vi "Launch Step Async.vi"(8 "error in (no error)":errorcluster, 10 "Step in":refnum<class "Step.lvclass">, 11 "Tester in":refnum<class "Tester.lvclass">) -> (0 "error out":errorcluster, 2 "Terminate":bool, 3 "Tester out":refnum<class "Tester.lvclass">)   [LabVIEW 2020, in "Tester.lvlib" / "Tester.lvclass"]
uses:
  Tester.lvclass
  Step/Step.lvclass
  Tester.lvclass/Tester.ctl
  Run Step Async.vi
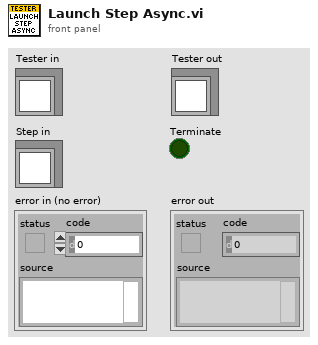
[diagram p1: front panel]
types:
  T1 = typedef "Tester.lvlib/Tester.lvclass/Execution Ref.ctl" = cluster{"Sequence":refnum<class "Sequence.lvclass">, "Step":i32, "Results":refnum<class "Results.lvclass">, "State":T2, "Run Step VI":refnum<vi>, "Abort":bool}
  T2 = typedef "Tester.lvlib/Tester.lvclass/State.ctl" = enum16{"Idle", "In Progress", "Completed"}
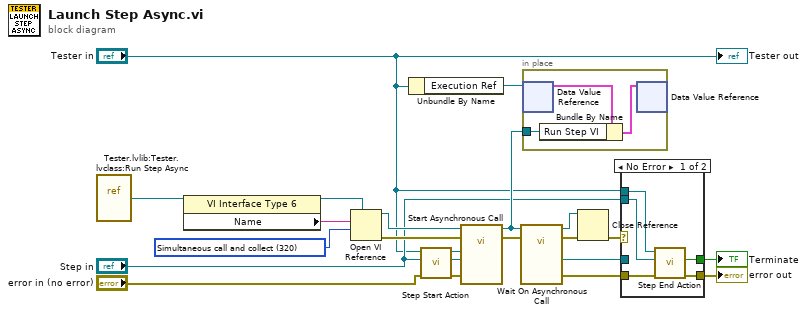
[diagram p0: block diagram]
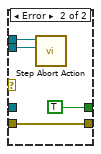
[diagram p2: hidden frame]
diagram:
  w19 = 320 items=["Record modifications"=1, "Open templates for editing"=2, "Prompt user to save"=4, "Prepare for reentrant run"=8, "Prompt to find missing subVIs"=16, "Hide loading dialog box"=32, "Enable simultaneous calls"=64, "Prepare to call and forget"=128, "Simultaneous call and forget"=192, "Prepare to call and collect"=256, "Simultaneous call and collect"=320]
  n1 = vi-ref "Tester.lvlib:Tester.lvclass:Run Step Async.vi"() -> (w17:refnum<vi>)
  n2 = property class="VI Interface Type 6"(reference=w17) -> (reference out=w20:refnum<vi>, "Name"=w18:string)  [unwired: 1 in, 1 out]
  n3 = Open VI Reference(type specifier VI Refnum (for type only)=w20, vi path=w18, options=w19) -> (vi reference=w22:refnum<vi>, error out=w21:errorcluster)  [unwired: 3 in]
  n4 = Unbundle By Name("Tester in") -> ("Execution Ref"=w16:refnum<data-value>)
  n5 = call-dynamic "Step Start Action.vi"("error in (no error)"="error in (no error)", "Step in"="Step in", "Tester in"="Tester in") -> ("error out"=w4:errorcluster, "Step out"=w5:refnum<class "Step.lvclass">, "Tester out"=w6:refnum<class "Tester.lvclass">)  [unwired: 6 in]
  n6 = call-by-ref "Start Asynchronous Call"(reference=w22, error in=w21, 8:"error in (no error)"=w4, "Step in"=w5, "Tester in"=w6) -> (reference out=w15:refnum<vi>, error out=w14:errorcluster)  [unwired: 7 in, 2 out]
  n7 = call-by-ref "Wait On Asynchronous Call"(reference=w15, error in=w14) -> (reference out=w12:refnum<vi>, error out=w13:errorcluster, 0:"error out"=w10:errorcluster, "Step out"=w9:refnum<class "Step.lvclass">)  [unwired: 10 in]
  n8 = in-place {
    in-place-border: w15 -> [w23]
    n9 = in-place-dvr #1(w16) -> (w25:T1)  [unwired: 1 out]
    n10 = Bundle By Name(cluster=w25, "Run Step VI"=w23) -> (w24:T1)
    n11 = in-place-dvr #1(w24) -> ()  [unwired: 2 out]
  }
  n12 = Close Reference(reference=w12, error in (no error)=w13) -> (error out=w11:errorcluster)
  n13 = case shown="No Error" w11 {
    tunnel: "Tester in" -> [w29 w34]
    tunnel: "Step in" -> [w28 w33]
    tunnel: w10 -> [w30 w31]
    tunnel: w9 -> [_ _]
    tunnel: [w27 w31] -> w8
    tunnel: [w26 TRUE ("Terminate")] -> w7
    frame No Error {
      n14 = call-dynamic "Step End Action.vi"("error in (no error)"=w30, "Step"=w28, "Tester in"=w29) -> ("error out"=w27:errorcluster, "Terminate"=w26:bool)  [unwired: 6 in, 1 out]
    }
    frame Error {
      n15 = call-dynamic "Step Abort Action.vi"("Step"=w33, "Tester in"=w34) -> ()  [unwired: 8 in, 2 out]
    }
  }
  "error out" <- w8
  "Terminate" <- w7
  "Tester out" <- "Tester in"
